vi "test PXI Chassis Clock Deployment.vi"(8 "error in (no error)":errorcluster, 11 "TestCase in":refnum<class "PharLap System Tests.lvclass">) -> (0 "error out":errorcluster, 3 "TestCase out":refnum<class "PharLap System Tests.lvclass">)   [LabVIEW 2015, in "PharLap System Tests.lvclass"]
uses:
  PharLap System Tests.lvclass
  <vilib>/addons/_JKI Toolkits/VI Tester/TestCase.llb/TestCase.lvclass
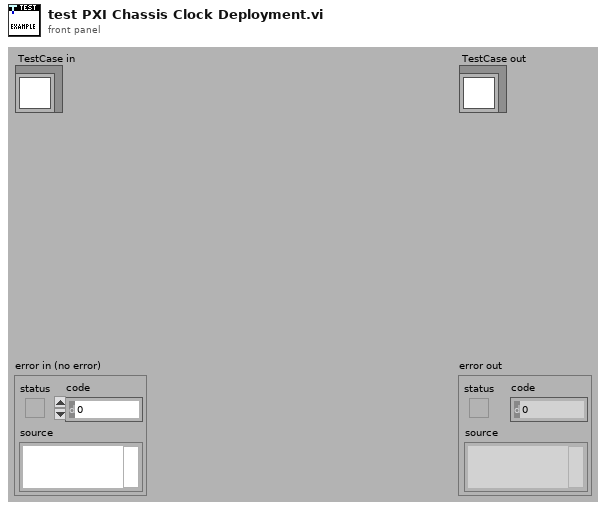
[diagram p1: front panel]
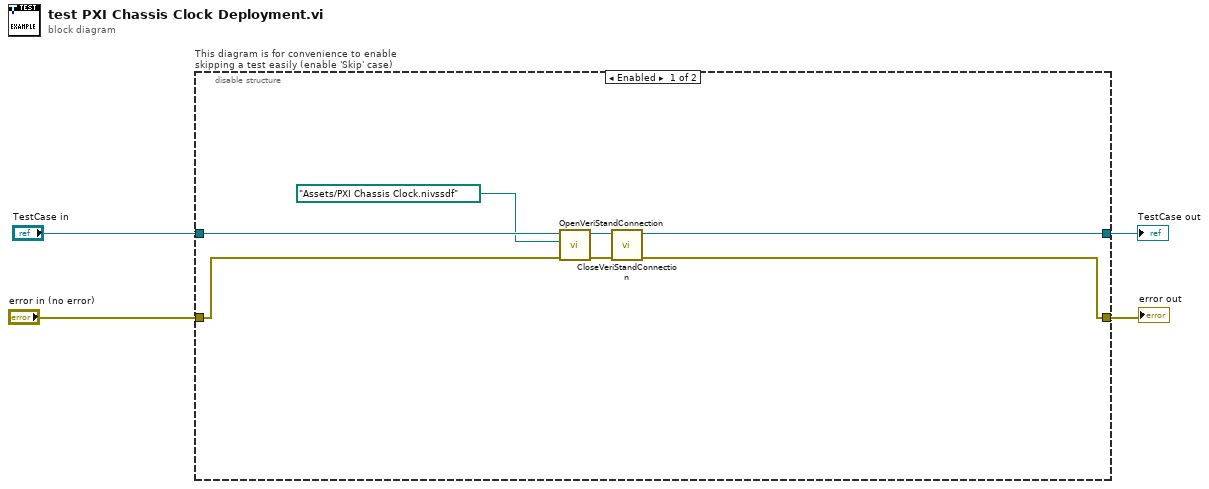
[diagram p0: block diagram]
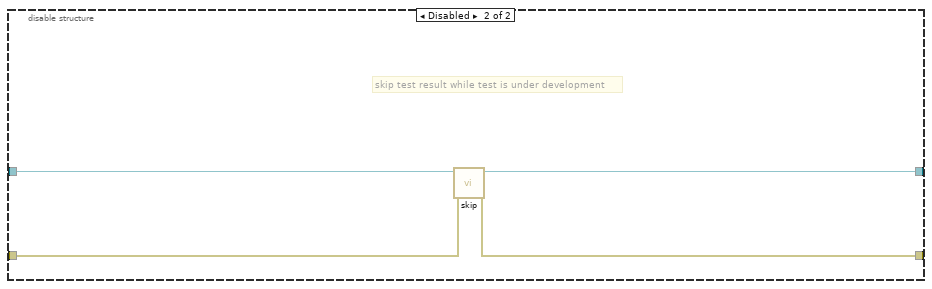
[diagram p2: hidden frame]
diagram:
  n1 = disable-structure "This diagram is for convenience to enable skipping a test easily (enable 'Skip' case)" shown="Enabled" {
    disable-tunnel: "TestCase in" -> [w11 w15]
    disable-tunnel: [w9 w13] -> w1
    disable-tunnel: [w6 w14] -> w3
    disable-tunnel: "error in (no error)" -> [w8 w12]
    frame Enabled {
      n2 = call-dynamic "OpenVeriStandConnection.vi"("error in (no error)"=w8, "System Definition File"=path "Assets/PXI Chassis Clock.nivssdf", "VeriStand Test Case in"=w11) -> ("error out"=w7:errorcluster, "VeriStand Test Case out"=w10:refnum<class "PharLap System Tests.lvclass">)  [unwired: 7 in]
      n3 = call-dynamic "CloseVeriStandConnection.vi"("error in (no error)"=w7, "VeriStand Test Case in"=w10) -> ("error out"=w6:errorcluster, "VeriStand Test Case out"=w9:refnum<class "PharLap System Tests.lvclass">)  [unwired: 8 in]
    }
    frame Disabled {
      # "skip test result while test is under development"
      n4 = call <vilib>:"skip.vi"("error in (no error)"=w12, "TestCase in"=w15) -> ("error out"=w14:errorcluster, "TestCase out"=w13:refnum<class "PharLap System Tests.lvclass">)  [unwired: 8 in]
    }
  }
  "error out" <- w3
  "TestCase out" <- w1
